vi "Find Window.vi"(8 "error in (no error)":errorcluster, 11 "Window Title (Callers Window)":string) -> (0 "error out":errorcluster, 3 "Window Handle":refnum<k24>)   [LabVIEW 2016, in "Progress Bar.lvclass"]
uses:
  <userlib>/_MGI/User Interface/Progress Bar/Progress Bar.lvclass
  kernel32.dll
  User32.dll
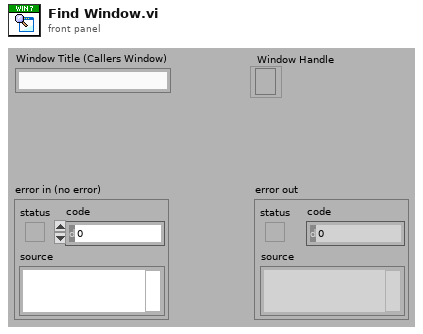
[diagram p1: front panel]
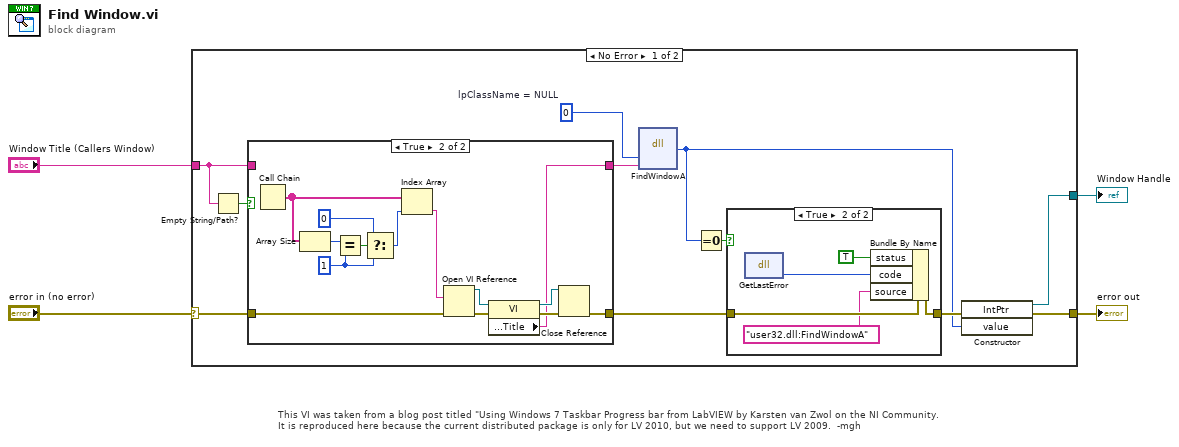
[diagram p0: block diagram]
diagram:
  # "This VI was taken from a blog post titled \"Using Windows 7 Taskbar Progress bar from LabVIEW by Karsten van Zwol on the NI Community.\nIt is reproduced here because the current distributed package is only for LV 2010, but we need to support LV 2009.  -mgh"
  n1 = case shown="No Error" "error in (no error)" {
    selector: "error in (no error)" -> [w10 w38]
    tunnel: [w7 w38] -> w3
    tunnel: "Window Title (Callers Window)" -> [w12 _]
    tunnel: [w5 _] -> w1
    frame No Error {
      w14 = u32 0  # lpClassName = NULL
      n2 = Empty String/Path?(string/path=w12) -> (empty?=w13:bool)
      n3 = case shown="True" w13 {
        tunnel: w12 -> [w17 _]
        tunnel: [w17 w19] -> w11
        tunnel: w10 -> [w16 w24]
        tunnel: [w16 w18] -> w9
        frame False {
        }
        frame True {
          w28 = 1 ("y")
          n4 = Call Chain() -> (call chain=w31:string[])
          n5 = Array Size(array=w31) -> (size(s)=w30:i32)
          n6 = Equal?(x=w30, y=w28) -> (x = y?=w29:bool)
          n7 = Select(t=0, s=w29, f=w28) -> (s? t:f=w26:i32)
          n8 = Index Array(array=w31, index=w26) -> (element=w25:string)
          n9 = Open VI Reference(vi path=w25, error in (no error)=w24) -> (vi reference=w22:refnum<vi>, error out=w23:errorcluster)  [unwired: 4 in]
          n10 = property class="VI"(reference=w22, error in=w23) -> (reference out=w20:refnum<vi>, error out=w21:errorcluster, "Front Panel.Title"=w19:string)
          n11 = Close Reference(reference=w20, error in (no error)=w21) -> (error out=w18:errorcluster)
        }
      }
      n12 = dll-call lib="user32.dll" fn="FindWindowA"("lpClassName"=w14, "lpWindowName"=w11) -> ("return type"=w6:i32)  [unwired: 5 in, 2 out]
      n13 = Equal To 0?(x=w6) -> (x = 0?=w15:bool)
      n14 = case shown="True" w15 {
        tunnel: [w32 w36] -> w8
        tunnel: w9 -> [w32 w37]
        frame False {
        }
        frame True {
          n15 = dll-call lib="kernel32.dll" fn="GetLastError"() -> ("return type"=w35:i32)  [unwired: 3 in, 2 out]
          n16 = Bundle By Name(cluster=w37, "status"=TRUE, "code"=w35, "source"="user32.dll:FindWindowA" ("Function")) -> (w36:errorcluster)
        }
      }
      n17 = constructor class="IntPtr"(error in=w8, "value"=w6) -> (reference out=w5:refnum<k24>, error out=w7:errorcluster)  [unwired: 2 in, 2 out]
    }
    frame Error {
    }
  }
  "error out" <- w3
  "Window Handle" <- w1
